vi "CBM_WriteBool_PLC_Keyence.vi"(8 "Set?":bool, 9 "MemoryNumber":string, 11 "PLC_IP":string) -> (2 "qBool":bool)   [LabVIEW 2017]
panel:
  out "error out":errorcluster
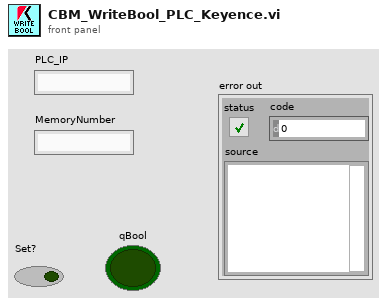
[diagram p1: front panel]
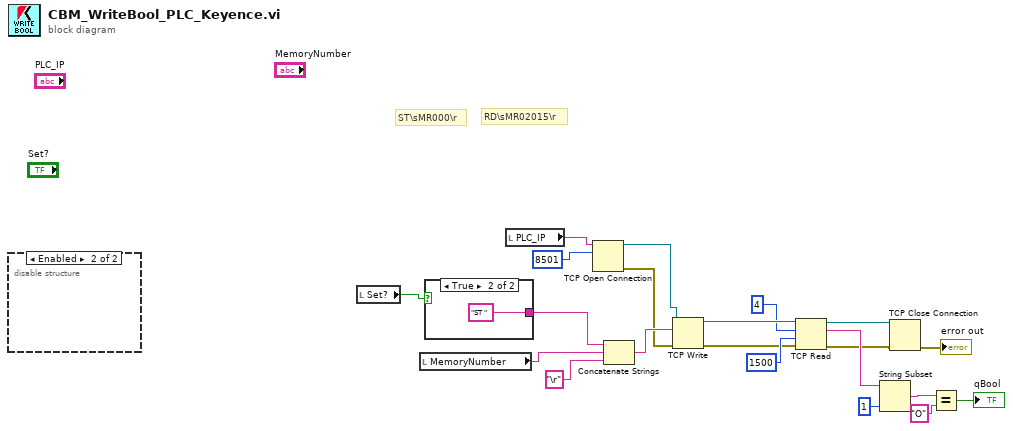
[diagram p0: block diagram]
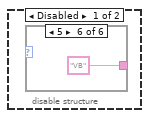
[diagram p2: hidden frame]
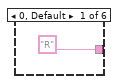
[diagram p3: hidden frame]
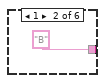
[diagram p4: hidden frame]
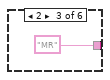
[diagram p5: hidden frame]
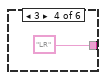
[diagram p6: hidden frame]
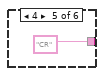
[diagram p7: hidden frame]
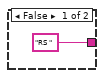
[diagram p8: hidden frame]
diagram:
  # "ST\\sMR000\\r"
  # "RD\\sMR02015\\r"
  n1 = disable-structure shown="Enabled" {
    frame Disabled {
      n2 = case shown="5" {
        selector: _ -> [_ _ _ _ _ _]
        tunnel: ["R" ("string") "B" ("string") "MR" ("string") "LR" ("string") "CR" ("string") "VB" ("string")] -> _
        frame 0, Default {
        }
        frame 1 {
        }
        frame 2 {
        }
        frame 3 {
        }
        frame 4 {
        }
        frame 5 {
        }
      }
    }
    frame Enabled {
    }
  }
  n3 = local read "Set?"() -> (w11:bool)
  n4 = local read "MemoryNumber"() -> (w2:string)
  n5 = case shown="True" w11 {
    tunnel: ["RS " ("string") "ST " ("string")] -> w12
    frame False {
    }
    frame True {
    }
  }
  n6 = local read "PLC_IP"() -> (w6:string)
  n7 = TCP Open Connection(address=w6, remote port or service name=8501 ("timeout ms (25000)")) -> (connection ID=w3:refnum<k5>, error out=w4:errorcluster)  [unwired: 3 in]
  n8 = Concatenate Strings(w12, w2, "\r" ("string")) -> (w14:string)
  n9 = TCP Write(connection ID=w3, data in=w14, error in (no error)=w4) -> (connection ID out=w21:refnum<k5>, error out=w10:errorcluster)  [unwired: 1 in, 1 out]
  n10 = TCP Read(connection ID=w21, bytes to read=4, error in (no error)=w10, 9:1500 ("timeout ms (25000)")) -> (connection ID out=w8:refnum<k5>, data out=w18:string, error out=w9:errorcluster)  [unwired: 1 in]
  n11 = String Subset(string=w18, length (rest)=1 ("length (rest)")) -> (substring=w16:string)  [unwired: 1 in]
  n12 = TCP Close Connection(connection ID=w8, error in (no error)=w9) -> (error out=→"error out":errorcluster)  [unwired: 1 in, 1 out]
  n13 = Equal?(x=w16, y="O") -> (x = y?=→"qBool":bool)
